vi "WyjsciaPC.vi"(8 "Akcja":T2, 11 "Wejœcie":T1) -> (3 "Wyjœcie":T1)   [LabVIEW 2014]
uses:
  glownaMaszynaStanowVIs/AkcjaGFV.ctl
  WyjsciaVIs/WyjsciaParametry.ctl
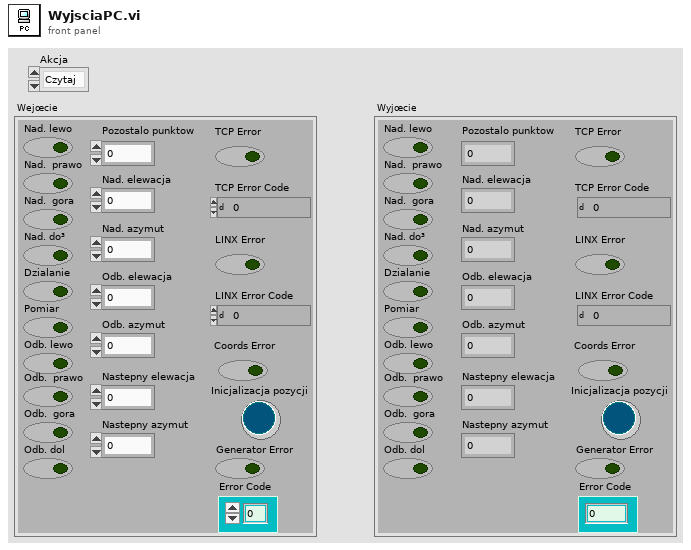
[diagram p1: front panel]
types:
  T1 = typedef "WyjsciaParametry.ctl" = cluster{"Nad. lewo":bool, "Nad.  prawo":bool, "Nad.  gora":bool, "Nad. do³":bool, "Dzialanie":bool, "Pomiar":bool, "Odb. lewo":bool, "Odb.  prawo":bool, "Odb.  gora":bool, "Odb. dol":bool, "Pozostalo punktow":i32, "Nad. elewacja":i32, "Nad. azymut":i32, "Odb. elewacja":i32, "Odb. azymut":i32, "TCP Error":bool, "TCP Error Code":i32, "LINX Error":bool, "LINX Error Code":i32, "Nastepny elewacja":i32, "Nastepny azymut":i32, "Coords Error":bool, "Inicjalizacja pozycji":bool, "Generator Error":bool, "Error Code":i32}
  T2 = typedef "AkcjaGFV.ctl" = enum16{"Czytaj", "Zapisz", "Reset"}
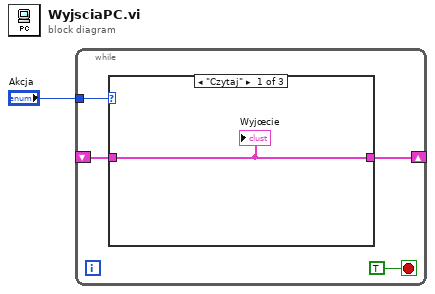
[diagram p0: block diagram]
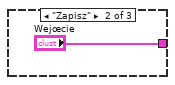
[diagram p2: hidden frame]
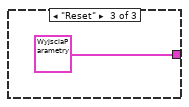
[diagram p3: hidden frame]
diagram:
  n1 = while {
    tunnel: "Akcja" -> [w4]
    shift-right: [w3] -> _
    shift-left: _ -> [w2]
    stop <- TRUE stop-if-true
    n2 = case shown="\"Czytaj\"" w4 {
      tunnel: [w6 "Wejœcie" T1 {"Nad. lewo"=FALSE, "Nad.  prawo"=FALSE, "Nad.  gora"=FALSE, "Nad. do³"=FALSE, "Dzialanie"=FALSE, "Pomiar"=FALSE, "Odb. lewo"=FALSE, "Odb.  prawo"=FALSE, "Odb.  gora"=FALSE, "Odb. dol"=FALSE, "Pozostalo punktow"=0, "Nad. elewacja"=0, "Nad. azymut"=0, "Odb. elewacja"=0, "Odb. azymut"=0, "TCP Error"=FALSE, "TCP Error Code"=0, "LINX Error"=FALSE, "LINX Error Code"=0, "Nastepny elewacja"=0, "Nastepny azymut"=0, "Coords Error"=FALSE, "Inicjalizacja pozycji"=FALSE, "Generator Error"=FALSE, "Error Code"=0} ("Cluster")] -> w3
      tunnel: w2 -> [w6 _ _]
      frame "Czytaj" {
        "Wyjœcie" <- w6
      }
      frame "Zapisz" {
      }
      frame "Reset" {
      }
    }
  }
